vi "Discover API.vi"(8 "error in (no error)":errorcluster, 10 "SMO":refnum<class "SMO.lvclass">) -> (0 "error out":errorcluster, 2 "PublicAPI":T1[](array[typedef]))   [LabVIEW 2021, in "smo.lvlib" / "Registry-SMO.lvclass"]
uses:
  Registry-SMO.lvclass
  SMO/SMO.lvclass
  SMO_API--Cluster.ctl
  SMOFacade/Terminal/Terminal.lvclass
  Registry-SMO.lvclass/Registry-SMO.ctl
  <vilib>/Utility/VariantDataType/VariantType.lvlib
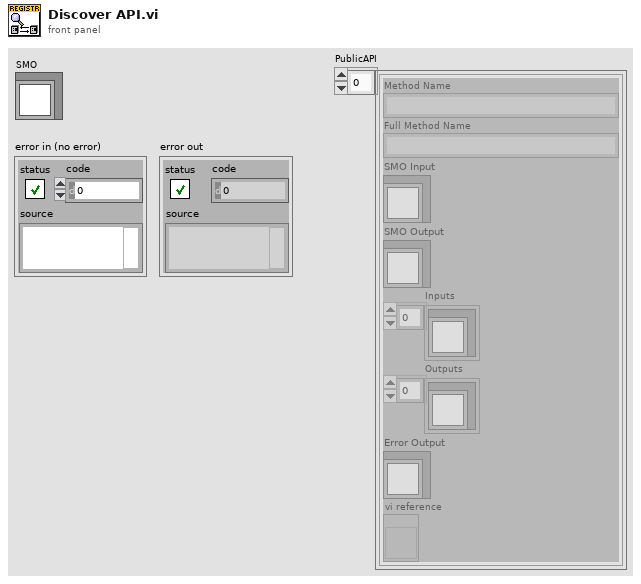
[diagram p1: front panel]
types:
  T1 = typedef "smo.lvlib/Registry-SMO.lvclass/SMO_API--Cluster.ctl" = cluster{"Method Name":string, "Full Method Name":string, "SMO Input":refnum<class "Terminal.lvclass">, "SMO Output":refnum<class "Terminal.lvclass">, "Inputs":refnum<class "Terminal.lvclass">[], "Outputs":refnum<class "Terminal.lvclass">[], "Error Output":refnum<class "Terminal.lvclass">, "vi reference":refnum<vi>}
  T2 = enum32{"invalid scope", "public", "private", "protected", "community"}
  T3 = typedef "VariantType.lvlib/VIInfo.ctl" = cluster{"Data1":i16, "Data2":i16, "Flags":u32[], "Modification Date":timestamp, "Asynchronous":bool, "NonFunctional":bool, "Subroutine":bool, "SubSystem":bool}
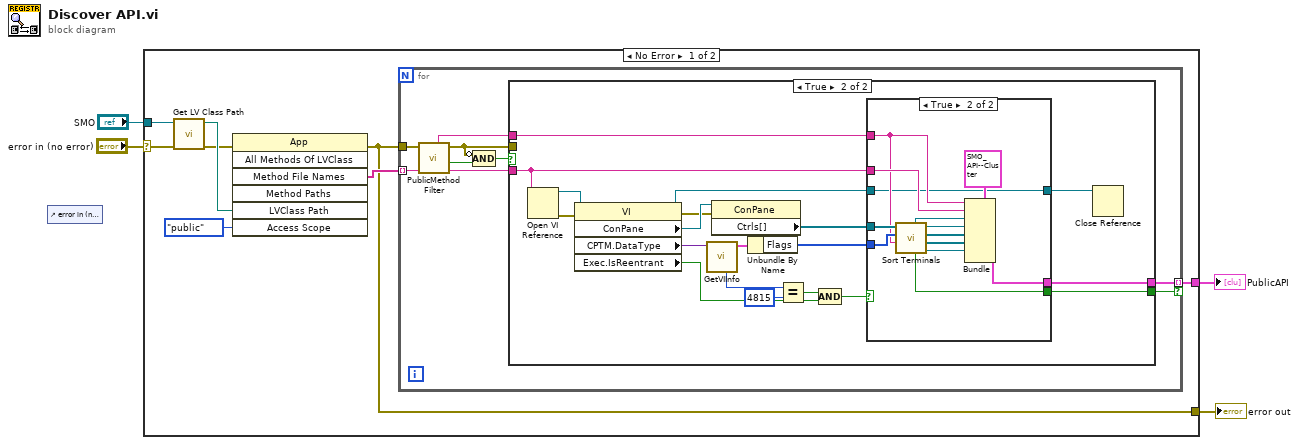
[diagram p0: block diagram]
diagram:
  n1 = control-ref of="error in (no error)"() -> ()  [unwired: 1 out]
  n2 = case shown="No Error" "error in (no error)" {
    selector: "error in (no error)" -> [w9 w55]
    tunnel: [w6 w55] -> w3
    tunnel: "SMO" -> [w12 _]
    tunnel: [w5 _] -> w1
    frame No Error {
      n3 = call <vilib>:"Get LV Class Path.vi"("error in (no error)"=w9, "object"=w12) -> ("error out"=w7:errorcluster, "class path"=w11:path)  [unwired: 8 in]
      n4 = invoke class="App" method="All Methods Of LVClass"(error in=w7, "LVClass Path"=w11, "Access Scope"=T2."public") -> (error out=w6:errorcluster, "Method File Names"=w8:string[])  [unwired: 4 in, 5 out]
      n5 = for {
        tunnel: w8 -> [w17] mode=indexing
        tunnel: [w21] -> w5 mode=indexing if=w20
        tunnel: w6 -> [w18]
        n6 = call "PublicMethod Filter.vi"("Full Method Name"=w17, "error in (no error)"=w18) -> ("Full Method Name dup"=w19:string, "Include?"=w16:bool, "error out"=w14:errorcluster, "Method Name"=w13:string)  [unwired: 6 in]
        n7 = Compound Arithmetic op=AND(invert w14, w16) -> (w15:bool)
        n8 = case shown="True" w15 {
          tunnel: [_ w40] -> w21
          tunnel: [_ w39] -> w20
          tunnel: w19 -> [_ w38]
          tunnel: w14 -> [_ _]
          tunnel: w13 -> [_ w37]
          frame False {
          }
          frame True {
            n9 = Open VI Reference(vi path=w38) -> (vi reference=w32:refnum<vi>, error out=w33:errorcluster)  [unwired: 5 in]
            n10 = property class="VI"(reference=w32, error in=w33) -> (reference out=w23:refnum<vi>, error out=w31:errorcluster, "ConPane"=w36:refnum<vi>, "CPTM.DataType"=w30:variant, "Exec.IsReentrant"=w24:bool)
            n11 = call <vilib>:"GetVIInfo.vi"("Variant"=w30) -> ("VI Info"=w28:T3, "pattern"=w29:i16)  [unwired: 6 in, 3 out]
            n12 = property class="ConPane"(reference=w36, error in=w31) -> ("Ctrls[]"=w35:refnum<vi>[])  [unwired: 2 out]
            n13 = Unbundle By Name(w28) -> ("Flags"=w27:u32[])
            n14 = Equal?(x=w29, y=i16 4815) -> (x = y?=w26:bool)
            n15 = Compound Arithmetic op=AND(w26, w24) -> (w25:bool)
            n16 = case shown="True" w25 {
              tunnel: [_ w44] -> w40
              tunnel: w35 -> [_ w52]
              tunnel: [_ w50] -> w39
              tunnel: w38 -> [_ w54]
              tunnel: w37 -> [_ w43]
              tunnel: w27 -> [_ w51]
              tunnel: w23 -> [w41 w42]
              tunnel: [w41 w42] -> w22
              frame False {
              }
              frame True {
                n17 = call "Sort Terminals.vi"("Method Name"=w43, "Flags"=w51, "Ctrls[]"=w52) -> ("Error Out"=w47:refnum<class "Terminal.lvclass">, "Outputs"=w45:refnum<class "Terminal.lvclass">[], "Inputs"=w46:refnum<class "Terminal.lvclass">[], "Operand Out"=w48:refnum<class "Terminal.lvclass">, "Valid API"=w50:bool, "Operand In"=w49:refnum<class "Terminal.lvclass">)  [unwired: 3 in]
                n18 = Bundle(cluster=T1 {"Method Name"="", "Full Method Name"="", "SMO Input"=refnum, "SMO Output"=refnum, "Inputs"=[], "Outputs"=[], "Error Output"=refnum, "vi reference"=refnum}, "Method Name"=w43, "Full Method Name"=w54, "SMO Input"=w49, "SMO Output"=w48, "Inputs"=w46, "Outputs"=w45, "Error Output"=w47) -> (w44:T1)  [unwired: 1 in]
              }
            }
            n19 = Close Reference(reference=w22) -> ()  [unwired: 1 in, 1 out]
          }
        }
      }
    }
    frame Error {
    }
  }
  "error out" <- w3
  "PublicAPI" <- w1
